vi "Configuration Data FGV.vi"   [LabVIEW 2014, in "LVH-KinectOne.lvlib"]
uses:
  LVH-KinectOne.lvlib
  Microsoft.Kinect
types:
  T1 = enum16{"ColorFrameDescription {Get}", "ColorFrameDescription {Set}", "DepthFrameDescription {Get}", "DepthFrameDescription {Set}", "InfraredFrameDescription {Get}", "InfraredFrameDescription {Set}"}
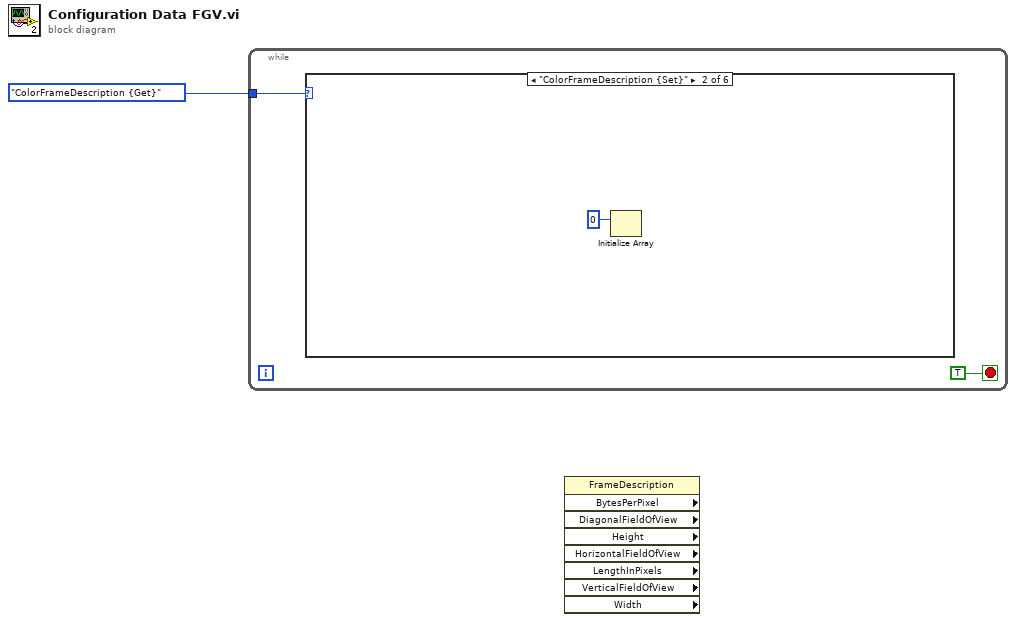
[diagram p0: block diagram]
diagram:
  n1 = while {
    tunnel: T1."ColorFrameDescription {Get}" -> [w3]
    stop <- TRUE stop-if-true
    n2 = case shown="\"ColorFrameDescription {Set}\"" w3 {
      frame "ColorFrameDescription {Get}", Default {
      }
      frame "ColorFrameDescription {Set}" {
        n3 = Initialize Array(u8 0) -> ()  [unwired: 1 in, 1 out]
      }
      frame "DepthFrameDescription {Get}" {
      }
      frame "DepthFrameDescription {Set}" {
      }
      frame "InfraredFrameDescription {Get}" {
      }
      frame "InfraredFrameDescription {Set}" {
      }
    }
  }
  n4 = property class="FrameDescription" props=["BytesPerPixel", "DiagonalFieldOfView", "Height", "HorizontalFieldOfView", "LengthInPixels", "VerticalFieldOfView", "Width"]() -> ()  [unwired: 2 in, 9 out]
